vi "Load Instrument Classes.vi"(8 "error in (no error)":errorcluster, 11 "Control Experiment.lvclass":refnum<class "Control Experiment.lvclass">) -> (0 "error out":errorcluster, 3 "Control Experiment out":refnum<class "Control Experiment.lvclass">)   [LabVIEW 2019, in "Control Experiment.lvclass"]
uses:
  Control Experiment.lvclass
  Control Experiment.lvclass/Control Experiment.ctl
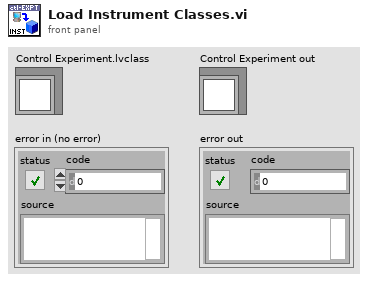
[diagram p1: front panel]
types:
  T1 = typedef "Control Experiment.lvclass/Instrument--enum.ctl" = enum16{"----- AFM/EBL -----", "AGILENT", "CYPHER", "Gemini2", "JEOL", "MFP3D", "----- Cryostat -----", "CF900", "DR200", "MNK", "PPMS (simulated)", "PPMS 1", "PPMS 2", "PPMS 3", "----- Optics -----", "THz 1 (Element 2/Montana)", "THz 2 (Tsunami/Janis)"}
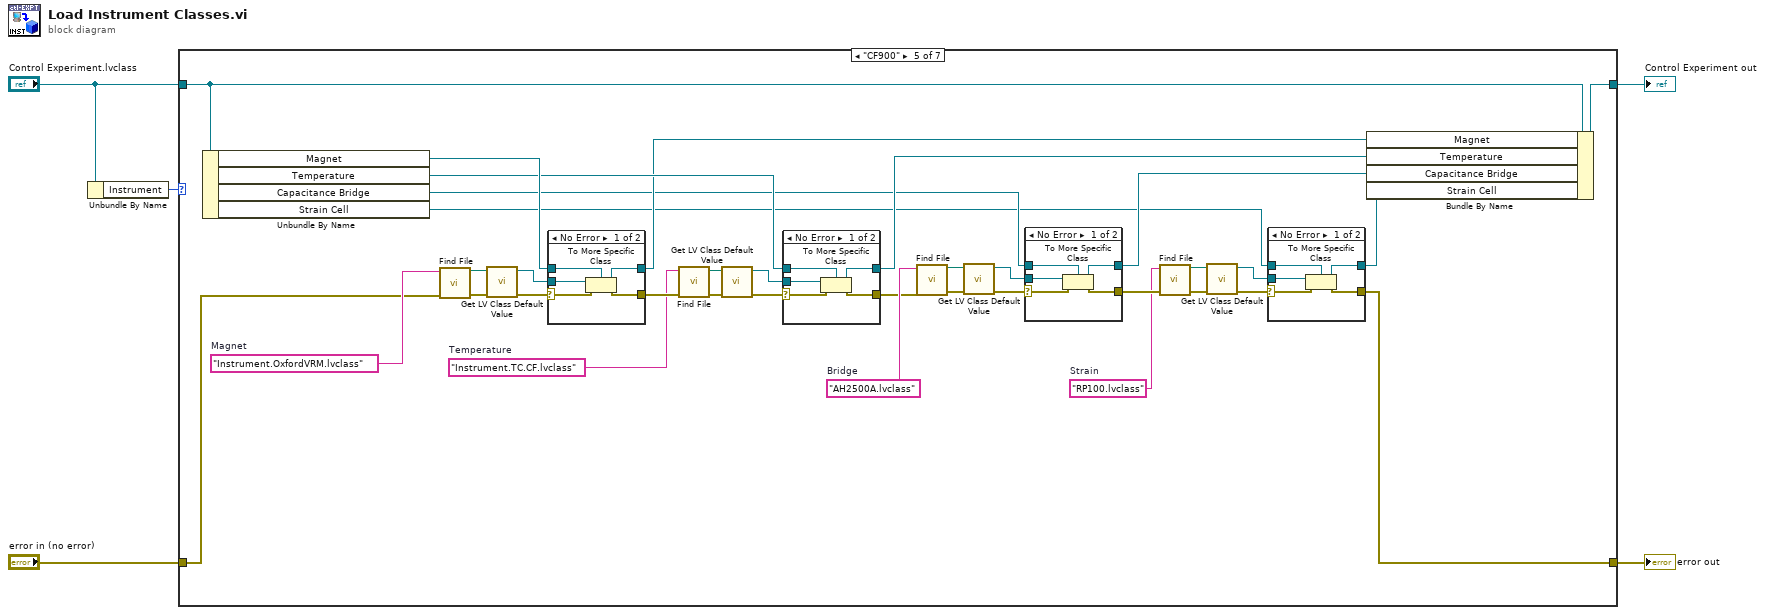
[diagram p0: block diagram]
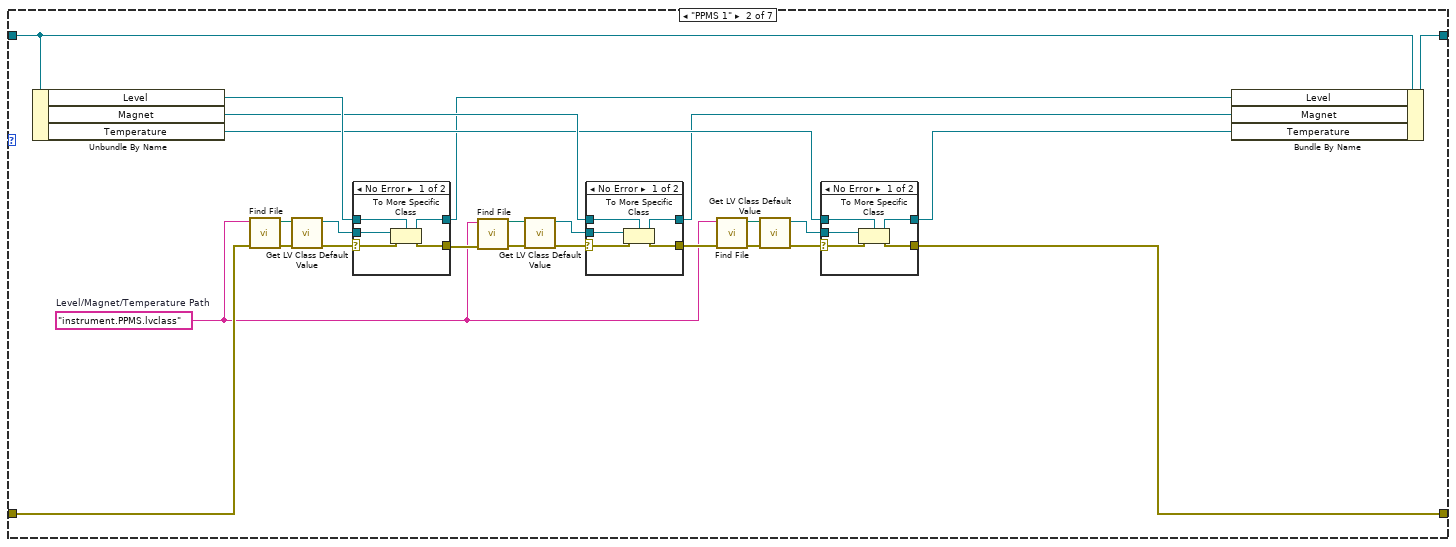
[diagram p3: hidden frame]
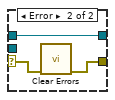
[diagram p4: hidden frame]
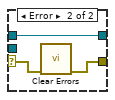
[diagram p5: hidden frame]
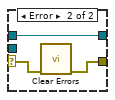
[diagram p6: hidden frame]
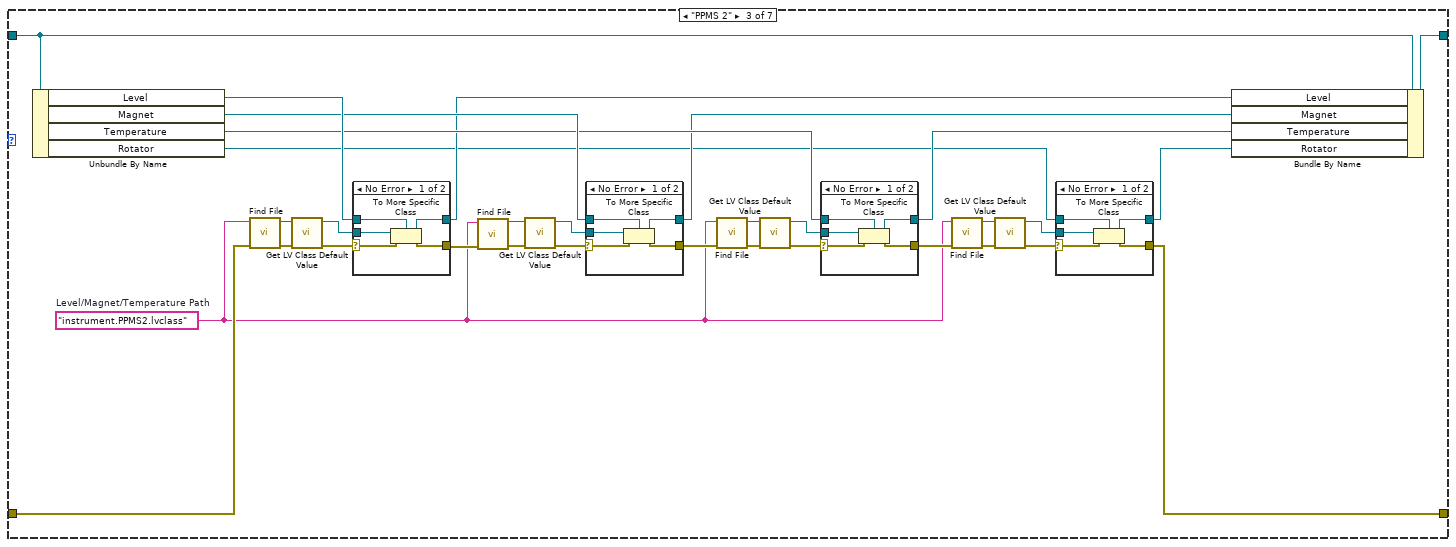
[diagram p7: hidden frame]
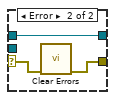
[diagram p8: hidden frame]
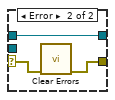
[diagram p9: hidden frame]
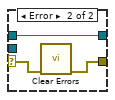
[diagram p10: hidden frame]
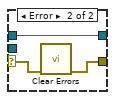
[diagram p11: hidden frame]
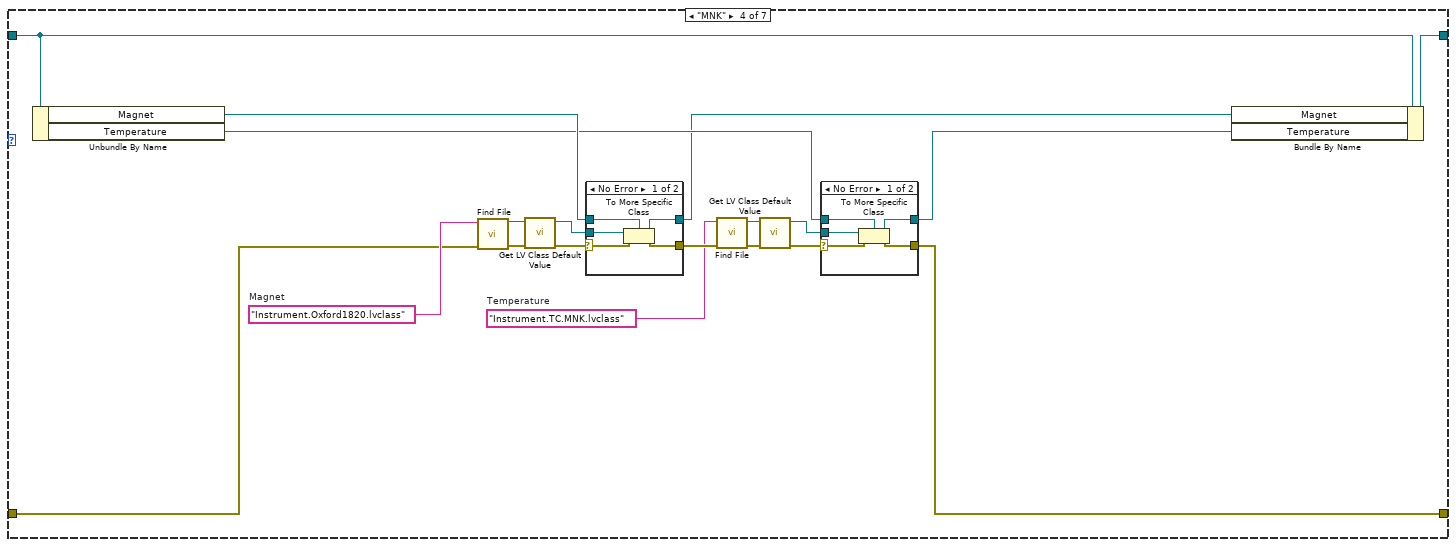
[diagram p12: hidden frame]
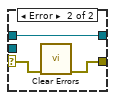
[diagram p13: hidden frame]
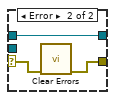
[diagram p14: hidden frame]
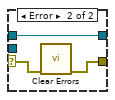
[diagram p15: hidden frame]
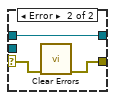
[diagram p16: hidden frame]
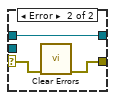
[diagram p17: hidden frame]
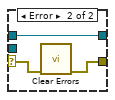
[diagram p18: hidden frame]
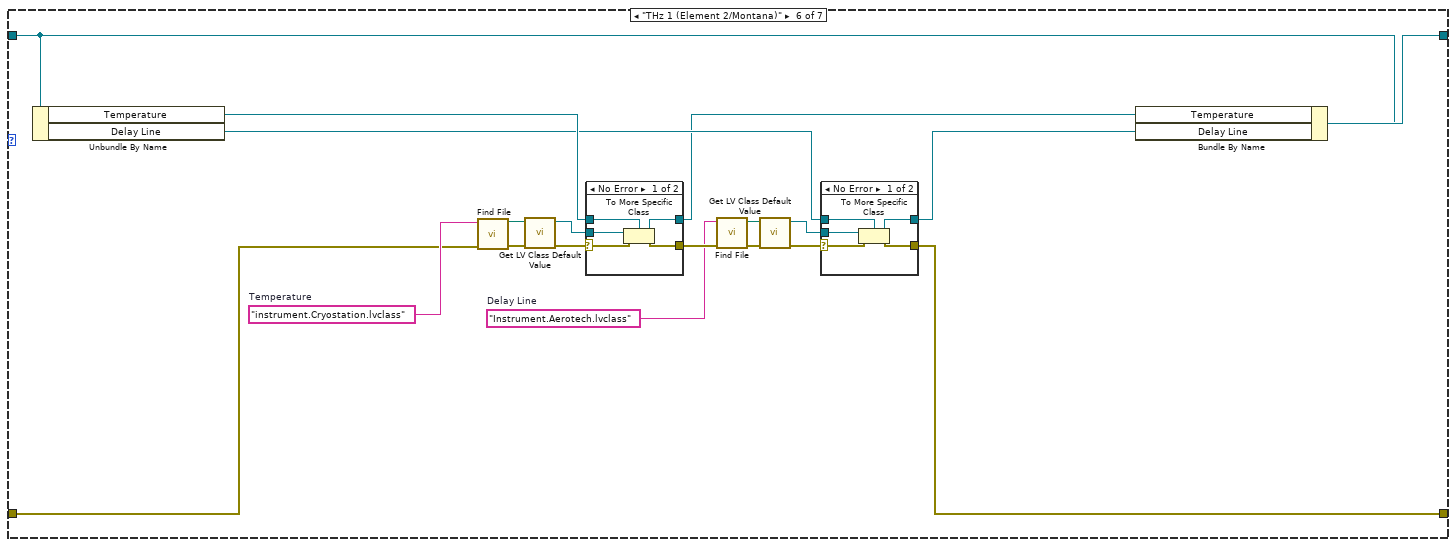
[diagram p19: hidden frame]
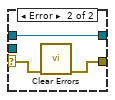
[diagram p20: hidden frame]
diagram:
  n1 = Unbundle By Name("Control Experiment.lvclass") -> ("Instrument"=w2:T1)
  n2 = case shown="\"CF900\"" w2 {
    tunnel: [w6 w18 w58 w121 w156 w223 w258] -> w5
    tunnel: [w7 w32 w88 w139 w190 w241 w284] -> w4
    tunnel: "Control Experiment.lvclass" -> [w7 w31 w87 w138 w189 w240 w283]
    tunnel: "error in (no error)" -> [w6 w17 w74 w122 w173 w224 w275]
    frame Default {
    }
    frame "PPMS 1" {
      w8 = "instrument.PPMS.lvclass"  # Level/Magnet/Temperature Path
      n3 = Unbundle By Name(w31) -> ("Level"=w28:refnum<class "Instrument.Cryostat.lvclass">, "Magnet"=w23:refnum<class "Instrument.Cryostat.lvclass">, "Temperature"=w22:refnum<class "Instrument.Cryostat.lvclass">)
      n4 = call "Find File.vi"("error in (no error)"=w17, "File Name"=w8) -> ("error out"=w19:errorcluster, "Path"=w15:path)  [unwired: 8 in]
      n5 = call <vilib>:"Get LV Class Default Value.vi"("error in (no error)"=w19, "class path"=w15) -> ("error out"=w29:errorcluster, "object"=w30:refnum<class>)  [unwired: 8 in]
      n6 = case shown="No Error" w29 {
        selector: w29 -> [w43 w46]
        tunnel: [w41 w47] -> w16
        tunnel: w30 -> [w45 _]
        tunnel: [w44 w48] -> w12
        tunnel: w28 -> [w42 w47]
        frame No Error {
          n7 = To More Specific Class(target class=w42, reference=w45, error in=w43) -> (specific class reference=w41:refnum<class "Instrument.Cryostat.lvclass">, error out=w44:errorcluster)
        }
        frame Error {
          n8 = call <vilib>:"Clear Errors.vi"("error in (no error)"=w46) -> ("error out"=w48:errorcluster)  [unwired: 5 in, 1 out]
        }
      }
      n9 = call "Find File.vi"("error in (no error)"=w12, "File Name"=w8) -> ("error out"=w14:errorcluster, "Path"=w13:path)  [unwired: 8 in]
      n10 = call <vilib>:"Get LV Class Default Value.vi"("error in (no error)"=w14, "class path"=w13) -> ("error out"=w27:errorcluster, "object"=w26:refnum<class>)  [unwired: 8 in]
      n11 = case shown="No Error" w27 {
        selector: w27 -> [w35 w38]
        tunnel: [w33 w39] -> w20
        tunnel: w26 -> [w37 _]
        tunnel: [w36 w40] -> w9
        tunnel: w23 -> [w34 w39]
        frame No Error {
          n12 = To More Specific Class(target class=w34, reference=w37, error in=w35) -> (specific class reference=w33:refnum<class "Instrument.Cryostat.lvclass">, error out=w36:errorcluster)
        }
        frame Error {
          n13 = call <vilib>:"Clear Errors.vi"("error in (no error)"=w38) -> ("error out"=w40:errorcluster)  [unwired: 5 in, 1 out]
        }
      }
      n14 = call "Find File.vi"("error in (no error)"=w9, "File Name"=w8) -> ("error out"=w11:errorcluster, "Path"=w10:path)  [unwired: 8 in]
      n15 = call <vilib>:"Get LV Class Default Value.vi"("error in (no error)"=w11, "class path"=w10) -> ("error out"=w24:errorcluster, "object"=w25:refnum<class>)  [unwired: 8 in]
      n16 = case shown="No Error" w24 {
        selector: w24 -> [w51 w54]
        tunnel: [w49 w55] -> w21
        tunnel: w25 -> [w53 _]
        tunnel: [w52 w56] -> w18
        tunnel: w22 -> [w50 w55]
        frame No Error {
          n17 = To More Specific Class(target class=w50, reference=w53, error in=w51) -> (specific class reference=w49:refnum<class "Instrument.Cryostat.lvclass">, error out=w52:errorcluster)
        }
        frame Error {
          n18 = call <vilib>:"Clear Errors.vi"("error in (no error)"=w54) -> ("error out"=w56:errorcluster)  [unwired: 5 in, 1 out]
        }
      }
      n19 = Bundle By Name(cluster=w31, "Level"=w16, "Magnet"=w20, "Temperature"=w21) -> (w32:refnum<class "Control Experiment.lvclass">)
    }
    frame "PPMS 2" {
      w57 = "instrument.PPMS2.lvclass"  # Level/Magnet/Temperature Path
      n20 = Unbundle By Name(w87) -> ("Level"=w84:refnum<class "Instrument.Cryostat.lvclass">, "Magnet"=w79:refnum<class "Instrument.Cryostat.lvclass">, "Temperature"=w78:refnum<class "Instrument.Cryostat.lvclass">, "Rotator"=w60:refnum<class "Instrument.Cryostat.lvclass">)
      n21 = call "Find File.vi"("error in (no error)"=w74, "File Name"=w57) -> ("error out"=w75:errorcluster, "Path"=w72:path)  [unwired: 8 in]
      n22 = call <vilib>:"Get LV Class Default Value.vi"("error in (no error)"=w75, "class path"=w72) -> ("error out"=w85:errorcluster, "object"=w86:refnum<class>)  [unwired: 8 in]
      n23 = case shown="No Error" w85 {
        selector: w85 -> [w107 w110]
        tunnel: [w105 w111] -> w73
        tunnel: w86 -> [w109 _]
        tunnel: [w108 w112] -> w69
        tunnel: w84 -> [w106 w111]
        frame No Error {
          n24 = To More Specific Class(target class=w106, reference=w109, error in=w107) -> (specific class reference=w105:refnum<class "Instrument.Cryostat.lvclass">, error out=w108:errorcluster)
        }
        frame Error {
          n25 = call <vilib>:"Clear Errors.vi"("error in (no error)"=w110) -> ("error out"=w112:errorcluster)  [unwired: 5 in, 1 out]
        }
      }
      n26 = call "Find File.vi"("error in (no error)"=w69, "File Name"=w57) -> ("error out"=w71:errorcluster, "Path"=w70:path)  [unwired: 8 in]
      n27 = call <vilib>:"Get LV Class Default Value.vi"("error in (no error)"=w71, "class path"=w70) -> ("error out"=w83:errorcluster, "object"=w82:refnum<class>)  [unwired: 8 in]
      n28 = case shown="No Error" w83 {
        selector: w83 -> [w99 w102]
        tunnel: [w97 w103] -> w76
        tunnel: w82 -> [w101 _]
        tunnel: [w100 w104] -> w66
        tunnel: w79 -> [w98 w103]
        frame No Error {
          n29 = To More Specific Class(target class=w98, reference=w101, error in=w99) -> (specific class reference=w97:refnum<class "Instrument.Cryostat.lvclass">, error out=w100:errorcluster)
        }
        frame Error {
          n30 = call <vilib>:"Clear Errors.vi"("error in (no error)"=w102) -> ("error out"=w104:errorcluster)  [unwired: 5 in, 1 out]
        }
      }
      n31 = call "Find File.vi"("error in (no error)"=w66, "File Name"=w57) -> ("error out"=w68:errorcluster, "Path"=w67:path)  [unwired: 8 in]
      n32 = call <vilib>:"Get LV Class Default Value.vi"("error in (no error)"=w68, "class path"=w67) -> ("error out"=w80:errorcluster, "object"=w81:refnum<class>)  [unwired: 8 in]
      n33 = case shown="No Error" w80 {
        selector: w80 -> [w115 w118]
        tunnel: [w113 w119] -> w77
        tunnel: w81 -> [w117 _]
        tunnel: [w116 w120] -> w61
        tunnel: w78 -> [w114 w119]
        frame No Error {
          n34 = To More Specific Class(target class=w114, reference=w117, error in=w115) -> (specific class reference=w113:refnum<class "Instrument.Cryostat.lvclass">, error out=w116:errorcluster)
        }
        frame Error {
          n35 = call <vilib>:"Clear Errors.vi"("error in (no error)"=w118) -> ("error out"=w120:errorcluster)  [unwired: 5 in, 1 out]
        }
      }
      n36 = call "Find File.vi"("error in (no error)"=w61, "File Name"=w57) -> ("error out"=w64:errorcluster, "Path"=w65:path)  [unwired: 8 in]
      n37 = call <vilib>:"Get LV Class Default Value.vi"("error in (no error)"=w64, "class path"=w65) -> ("error out"=w63:errorcluster, "object"=w62:refnum<class>)  [unwired: 8 in]
      n38 = case shown="No Error" w63 {
        selector: w63 -> [w91 w94]
        tunnel: [w89 w95] -> w59
        tunnel: w62 -> [w93 _]
        tunnel: [w92 w96] -> w58
        tunnel: w60 -> [w90 w95]
        frame No Error {
          n39 = To More Specific Class(target class=w90, reference=w93, error in=w91) -> (specific class reference=w89:refnum<class "Instrument.Cryostat.lvclass">, error out=w92:errorcluster)
        }
        frame Error {
          n40 = call <vilib>:"Clear Errors.vi"("error in (no error)"=w94) -> ("error out"=w96:errorcluster)  [unwired: 5 in, 1 out]
        }
      }
      n41 = Bundle By Name(cluster=w87, "Level"=w73, "Magnet"=w76, "Temperature"=w77, "Rotator"=w59) -> (w88:refnum<class "Control Experiment.lvclass">)
    }
    frame "MNK" {
      w124 = "Instrument.TC.MNK.lvclass"  # Temperature
      w123 = "Instrument.Oxford1820.lvclass"  # Magnet
      n42 = Unbundle By Name(w138) -> ("Magnet"=w133:refnum<class "Instrument.Cryostat.lvclass">, "Temperature"=w132:refnum<class "Instrument.Cryostat.lvclass">)
      n43 = call "Find File.vi"("error in (no error)"=w122, "File Name"=w123) -> ("error out"=w129:errorcluster, "Path"=w128:path)  [unwired: 8 in]
      n44 = call <vilib>:"Get LV Class Default Value.vi"("error in (no error)"=w129, "class path"=w128) -> ("error out"=w137:errorcluster, "object"=w136:refnum<class>)  [unwired: 8 in]
      n45 = case shown="No Error" w137 {
        selector: w137 -> [w142 w145]
        tunnel: [w140 w146] -> w130
        tunnel: w136 -> [w144 _]
        tunnel: [w143 w147] -> w125
        tunnel: w133 -> [w141 w146]
        frame No Error {
          n46 = To More Specific Class(target class=w141, reference=w144, error in=w142) -> (specific class reference=w140:refnum<class "Instrument.Cryostat.lvclass">, error out=w143:errorcluster)
        }
        frame Error {
          n47 = call <vilib>:"Clear Errors.vi"("error in (no error)"=w145) -> ("error out"=w147:errorcluster)  [unwired: 5 in, 1 out]
        }
      }
      n48 = call "Find File.vi"("error in (no error)"=w125, "File Name"=w124) -> ("error out"=w127:errorcluster, "Path"=w126:path)  [unwired: 8 in]
      n49 = call <vilib>:"Get LV Class Default Value.vi"("error in (no error)"=w127, "class path"=w126) -> ("error out"=w134:errorcluster, "object"=w135:refnum<class>)  [unwired: 8 in]
      n50 = case shown="No Error" w134 {
        selector: w134 -> [w150 w153]
        tunnel: [w148 w154] -> w131
        tunnel: w135 -> [w152 _]
        tunnel: [w151 w155] -> w121
        tunnel: w132 -> [w149 w154]
        frame No Error {
          n51 = To More Specific Class(target class=w149, reference=w152, error in=w150) -> (specific class reference=w148:refnum<class "Instrument.Cryostat.lvclass">, error out=w151:errorcluster)
        }
        frame Error {
          n52 = call <vilib>:"Clear Errors.vi"("error in (no error)"=w153) -> ("error out"=w155:errorcluster)  [unwired: 5 in, 1 out]
        }
      }
      n53 = Bundle By Name(cluster=w138, "Magnet"=w130, "Temperature"=w131) -> (w139:refnum<class "Control Experiment.lvclass">)
    }
    frame "CF900" {
      w163 = "RP100.lvclass"  # Strain
      w162 = "AH2500A.lvclass"  # Bridge
      w175 = "Instrument.TC.CF.lvclass"  # Temperature
      w174 = "Instrument.OxfordVRM.lvclass"  # Magnet
      n54 = Unbundle By Name(w189) -> ("Magnet"=w184:refnum<class "Instrument.Cryostat.lvclass">, "Temperature"=w183:refnum<class "Instrument.Cryostat.lvclass">, "Capacitance Bridge"=w159:refnum<class "Instrument.CBridge.lvclass">, "Strain Cell"=w158:refnum<class "Instrument.Strain.lvclass">)
      n55 = call "Find File.vi"("error in (no error)"=w173, "File Name"=w174) -> ("error out"=w180:errorcluster, "Path"=w179:path)  [unwired: 8 in]
      n56 = call <vilib>:"Get LV Class Default Value.vi"("error in (no error)"=w180, "class path"=w179) -> ("error out"=w188:errorcluster, "object"=w187:refnum<class>)  [unwired: 8 in]
      n57 = case shown="No Error" w188 {
        selector: w188 -> [w209 w212]
        tunnel: [w207 w213] -> w181
        tunnel: w187 -> [w211 _]
        tunnel: [w210 w214] -> w176
        tunnel: w184 -> [w208 w213]
        frame No Error {
          n58 = To More Specific Class(target class=w208, reference=w211, error in=w209) -> (specific class reference=w207:refnum<class "Instrument.Cryostat.lvclass">, error out=w210:errorcluster)
        }
        frame Error {
          n59 = call <vilib>:"Clear Errors.vi"("error in (no error)"=w212) -> ("error out"=w214:errorcluster)  [unwired: 5 in, 1 out]
        }
      }
      n60 = call "Find File.vi"("error in (no error)"=w176, "File Name"=w175) -> ("error out"=w178:errorcluster, "Path"=w177:path)  [unwired: 8 in]
      n61 = call <vilib>:"Get LV Class Default Value.vi"("error in (no error)"=w178, "class path"=w177) -> ("error out"=w185:errorcluster, "object"=w186:refnum<class>)  [unwired: 8 in]
      n62 = case shown="No Error" w185 {
        selector: w185 -> [w217 w220]
        tunnel: [w215 w221] -> w182
        tunnel: w186 -> [w219 _]
        tunnel: [w218 w222] -> w157
        tunnel: w183 -> [w216 w221]
        frame No Error {
          n63 = To More Specific Class(target class=w216, reference=w219, error in=w217) -> (specific class reference=w215:refnum<class "Instrument.Cryostat.lvclass">, error out=w218:errorcluster)
        }
        frame Error {
          n64 = call <vilib>:"Clear Errors.vi"("error in (no error)"=w220) -> ("error out"=w222:errorcluster)  [unwired: 5 in, 1 out]
        }
      }
      n65 = call "Find File.vi"("error in (no error)"=w157, "File Name"=w162) -> ("error out"=w171:errorcluster, "Path"=w172:path)  [unwired: 8 in]
      n66 = call <vilib>:"Get LV Class Default Value.vi"("error in (no error)"=w171, "class path"=w172) -> ("error out"=w169:errorcluster, "object"=w170:refnum<class>)  [unwired: 8 in]
      n67 = case shown="No Error" w169 {
        selector: w169 -> [w201 w204]
        tunnel: [w199 w205] -> w160
        tunnel: w170 -> [w203 _]
        tunnel: [w202 w206] -> w164
        tunnel: w159 -> [w200 w205]
        frame No Error {
          n68 = To More Specific Class(target class=w200, reference=w203, error in=w201) -> (specific class reference=w199:refnum<class "Instrument.CBridge.lvclass">, error out=w202:errorcluster)
        }
        frame Error {
          n69 = call <vilib>:"Clear Errors.vi"("error in (no error)"=w204) -> ("error out"=w206:errorcluster)  [unwired: 5 in, 1 out]
        }
      }
      n70 = call "Find File.vi"("error in (no error)"=w164, "File Name"=w163) -> ("error out"=w166:errorcluster, "Path"=w165:path)  [unwired: 8 in]
      n71 = call <vilib>:"Get LV Class Default Value.vi"("error in (no error)"=w166, "class path"=w165) -> ("error out"=w168:errorcluster, "object"=w167:refnum<class>)  [unwired: 8 in]
      n72 = case shown="No Error" w168 {
        selector: w168 -> [w193 w196]
        tunnel: [w191 w197] -> w161
        tunnel: w167 -> [w195 _]
        tunnel: [w194 w198] -> w156
        tunnel: w158 -> [w192 w197]
        frame No Error {
          n73 = To More Specific Class(target class=w192, reference=w195, error in=w193) -> (specific class reference=w191:refnum<class "Instrument.Strain.lvclass">, error out=w194:errorcluster)
        }
        frame Error {
          n74 = call <vilib>:"Clear Errors.vi"("error in (no error)"=w196) -> ("error out"=w198:errorcluster)  [unwired: 5 in, 1 out]
        }
      }
      n75 = Bundle By Name(cluster=w189, "Magnet"=w181, "Temperature"=w182, "Capacitance Bridge"=w160, "Strain Cell"=w161) -> (w190:refnum<class "Control Experiment.lvclass">)
    }
    frame "THz 1 (Element 2/Montana)" {
      w226 = "Instrument.Aerotech.lvclass"  # Delay Line
      w225 = "instrument.Cryostation.lvclass"  # Temperature
      n76 = Unbundle By Name(w240) -> ("Temperature"=w235:refnum<class "Instrument.Cryostat.lvclass">, "Delay Line"=w234:refnum<class "Instrument.DelayLine.lvclass">)
      n77 = call "Find File.vi"("error in (no error)"=w224, "File Name"=w225) -> ("error out"=w231:errorcluster, "Path"=w230:path)  [unwired: 8 in]
      n78 = call <vilib>:"Get LV Class Default Value.vi"("error in (no error)"=w231, "class path"=w230) -> ("error out"=w239:errorcluster, "object"=w238:refnum<class>)  [unwired: 8 in]
      n79 = case shown="No Error" w239 {
        selector: w239 -> [w244 w247]
        tunnel: [w242 w248] -> w232
        tunnel: w238 -> [w246 _]
        tunnel: [w245 w249] -> w227
        tunnel: w235 -> [w243 w248]
        frame No Error {
          n80 = To More Specific Class(target class=w243, reference=w246, error in=w244) -> (specific class reference=w242:refnum<class "Instrument.Cryostat.lvclass">, error out=w245:errorcluster)
        }
        frame Error {
          n81 = call <vilib>:"Clear Errors.vi"("error in (no error)"=w247) -> ("error out"=w249:errorcluster)  [unwired: 5 in, 1 out]
        }
      }
      n82 = call "Find File.vi"("error in (no error)"=w227, "File Name"=w226) -> ("error out"=w229:errorcluster, "Path"=w228:path)  [unwired: 8 in]
      n83 = call <vilib>:"Get LV Class Default Value.vi"("error in (no error)"=w229, "class path"=w228) -> ("error out"=w236:errorcluster, "object"=w237:refnum<class>)  [unwired: 8 in]
      n84 = case shown="No Error" w236 {
        selector: w236 -> [w253 w255]
        tunnel: [w251 w256] -> w233
        tunnel: w237 -> [w250 _]
        tunnel: [w254 w257] -> w223
        tunnel: w234 -> [w252 w256]
        frame No Error {
          n85 = To More Specific Class(target class=w252, reference=w250, error in=w253) -> (specific class reference=w251:refnum<class "Instrument.DelayLine.lvclass">, error out=w254:errorcluster)
        }
        frame Error {
          n86 = call <vilib>:"Clear Errors.vi"("error in (no error)"=w255) -> ("error out"=w257:errorcluster)  [unwired: 5 in, 1 out]
        }
      }
      n87 = Bundle By Name(cluster=w240, "Temperature"=w232, "Delay Line"=w233) -> (w241:refnum<class "Control Experiment.lvclass">)
    }
    frame "DR200" {
      w261 = "RP100.lvclass"  # Strain
      w269 = "AH2500A.lvclass"  # Bridge
      w276 = "IPS120.lvclass"  # Magnet
      n88 = Unbundle By Name(w283) -> ("Magnet"=w280:refnum<class "Instrument.Cryostat.lvclass">, "Capacitance Bridge"=w267:refnum<class "Instrument.CBridge.lvclass">, "Strain Cell"=w260:refnum<class "Instrument.Strain.lvclass">)
      n89 = call "Find File.vi"("error in (no error)"=w275, "File Name"=w276) -> ("error out"=w278:errorcluster, "Path"=w277:path)  [unwired: 8 in]
      n90 = call <vilib>:"Get LV Class Default Value.vi"("error in (no error)"=w278, "class path"=w277) -> ("error out"=w282:errorcluster, "object"=w281:refnum<class>)  [unwired: 8 in]
      n91 = case shown="No Error" w282 {
        selector: w282 -> [w303 w306]
        tunnel: [w301 w307] -> w279
        tunnel: w281 -> [w305 _]
        tunnel: [w304 w308] -> w270
        tunnel: w280 -> [w302 w307]
        frame No Error {
          n92 = To More Specific Class(target class=w302, reference=w305, error in=w303) -> (specific class reference=w301:refnum<class "Instrument.Cryostat.lvclass">, error out=w304:errorcluster)
        }
        frame Error {
          n93 = call <vilib>:"Clear Errors.vi"("error in (no error)"=w306) -> ("error out"=w308:errorcluster)  [unwired: 5 in, 1 out]
        }
      }
      n94 = call "Find File.vi"("error in (no error)"=w270, "File Name"=w269) -> ("error out"=w273:errorcluster, "Path"=w274:path)  [unwired: 8 in]
      n95 = call <vilib>:"Get LV Class Default Value.vi"("error in (no error)"=w273, "class path"=w274) -> ("error out"=w271:errorcluster, "object"=w272:refnum<class>)  [unwired: 8 in]
      n96 = case shown="No Error" w271 {
        selector: w271 -> [w295 w298]
        tunnel: [w293 w299] -> w268
        tunnel: w272 -> [w297 _]
        tunnel: [w296 w300] -> w262
        tunnel: w267 -> [w294 w299]
        frame No Error {
          n97 = To More Specific Class(target class=w294, reference=w297, error in=w295) -> (specific class reference=w293:refnum<class "Instrument.CBridge.lvclass">, error out=w296:errorcluster)
        }
        frame Error {
          n98 = call <vilib>:"Clear Errors.vi"("error in (no error)"=w298) -> ("error out"=w300:errorcluster)  [unwired: 5 in, 1 out]
        }
      }
      n99 = call "Find File.vi"("error in (no error)"=w262, "File Name"=w261) -> ("error out"=w264:errorcluster, "Path"=w263:path)  [unwired: 8 in]
      n100 = call <vilib>:"Get LV Class Default Value.vi"("error in (no error)"=w264, "class path"=w263) -> ("error out"=w266:errorcluster, "object"=w265:refnum<class>)  [unwired: 8 in]
      n101 = case shown="No Error" w266 {
        selector: w266 -> [w287 w290]
        tunnel: [w285 w291] -> w259
        tunnel: w265 -> [w289 _]
        tunnel: [w288 w292] -> w258
        tunnel: w260 -> [w286 w291]
        frame No Error {
          n102 = To More Specific Class(target class=w286, reference=w289, error in=w287) -> (specific class reference=w285:refnum<class "Instrument.Strain.lvclass">, error out=w288:errorcluster)
        }
        frame Error {
          n103 = call <vilib>:"Clear Errors.vi"("error in (no error)"=w290) -> ("error out"=w292:errorcluster)  [unwired: 5 in, 1 out]
        }
      }
      n104 = Bundle By Name(cluster=w283, "Magnet"=w279, "Capacitance Bridge"=w268, "Strain Cell"=w259) -> (w284:refnum<class "Control Experiment.lvclass">)
    }
  }
  "error out" <- w5
  "Control Experiment out" <- w4
